vi "joystick scaleNtransform.vi"(8 "robot field orientation (deg)":dbl, 9 "joystick values":dbl[](array[numeric]), 10 "use filed orientation":bool, 11 "reset field orientation":bool) -> (3 "Transformed joystick values":dbl[](array[numeric]))   [LabVIEW 2018]
uses:
  <vilib>/Analysis/coordinate.llb/2D Cartesian Coordinate Rotation (Scalar).vi
  reset gyro.vi
  <vilib>/Analysis/NI_AALPro.lvlib
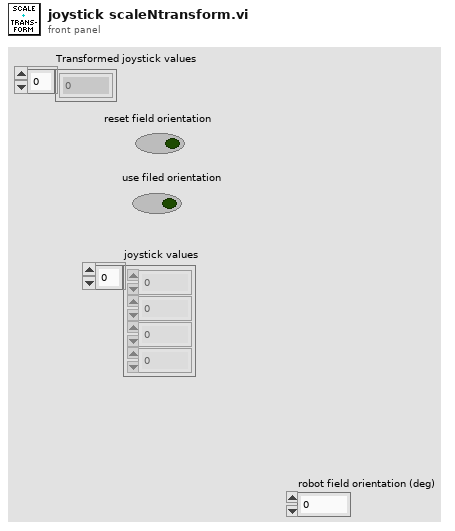
[diagram p1: front panel]
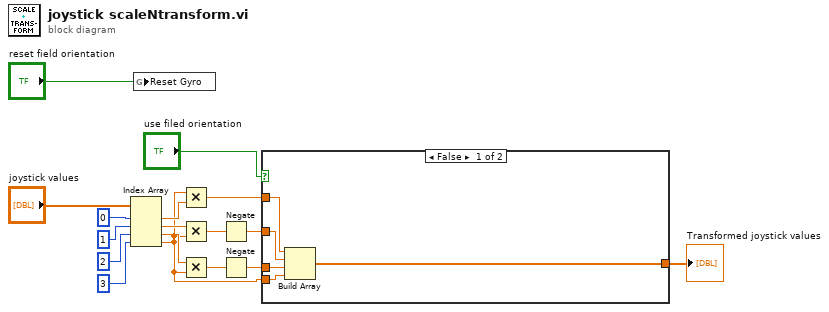
[diagram p0: block diagram]
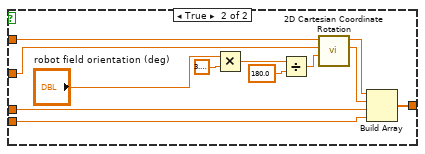
[diagram p2: hidden frame]
diagram:
  n1 = Index Array(array="joystick values", index #1=0 ("index"), index #2=1 ("index"), index #3=2 ("index"), index #4=3 ("index")) -> (element #1=w12:dbl, element #2=w11:dbl, element #3=w10:dbl, element #4=w3:dbl)
  n2 = global write "reset gyro.vi" "Reset Gyro"("reset field orientation") -> ()
  n3 = Multiply(x=w3, y=w12) -> (x*y=w6:dbl)
  n4 = Multiply(x=w11, y=w3) -> (x*y=w8:dbl)
  n5 = Multiply(x=w10, y=w3) -> (x*y=w7:dbl)
  n6 = Negate(x=w8) -> (-x=w5:dbl)
  n7 = Negate(x=w7) -> (-x=w4:dbl)
  n8 = case shown="False" "use filed orientation" {
    tunnel: w6 -> [w22 w34]
    tunnel: w5 -> [w21 w33]
    tunnel: w4 -> [w20 w25]
    tunnel: w3 -> [w19 w24]
    tunnel: [w18 w23] -> w1
    frame False {
      n9 = Build Array(w22, w21, w20, w19) -> (w18:dbl[])
    }
    frame True {
      n10 = Multiply(x="robot field orientation (deg)", y=3.141592653589793) -> (x*y=w30:dbl)
      n11 = Divide(x=w30, y=180.0) -> (x/y=w28:dbl)
      n12 = call-poly <vilib>:"2D Cartesian Coordinate Rotation.vi"("theta"=w28, "y"=w33, "x"=w34) -> ("y out"=w26:dbl, "x out"=w27:dbl)  [unwired: 6 in, 1 out]
      n13 = Build Array(w27, w26, w25, w24) -> (w23:dbl[])
    }
  }
  "Transformed joystick values" <- w1
